vi "Metadata_Creator.vi"(7 "Frame Timestamp":u64, 8 "error in (no error)":errorcluster, 9 "Frame Index":u32, 10 "EBD Config":T2, 11 "Image Data Config":T1={"Lines of Image Data"=0, "Bytes per Even Line"=0, "Bytes per Odd Line"=0, "Image Data Type"=44, "Total Image Data Block Size"=0, "Image Data Block Offset"=0} {"Image Data Type" format="%x"}) -> (0 "error out":errorcluster, 3 "Meta Data (U8)":u8[](array[numeric]))   [LabVIEW 2020]
uses:
  ctl/Image_EBD_Config.ctl
  ctl/Image_Data_Config.ctl
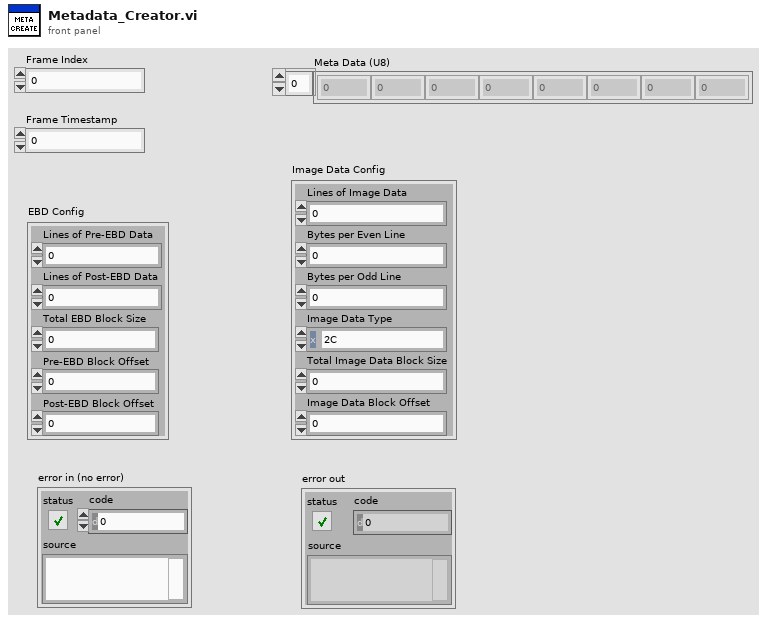
[diagram p1: front panel]
types:
  T1 = typedef "Image_Data_Config.ctl" = cluster{"Lines of Image Data":u16, "Bytes per Even Line":u16, "Bytes per Odd Line":u16, "Image Data Type":u8, "Total Image Data Block Size":u32, "Image Data Block Offset":u32}
  T2 = typedef "Image_EBD_Config.ctl" = cluster{"Lines of Pre-EBD Data":u16, "Lines of Post-EBD Data":u16, "Total EBD Block Size":u32, "Pre-EBD Block Offset ":u32, "Post-EBD Block Offset ":u32}
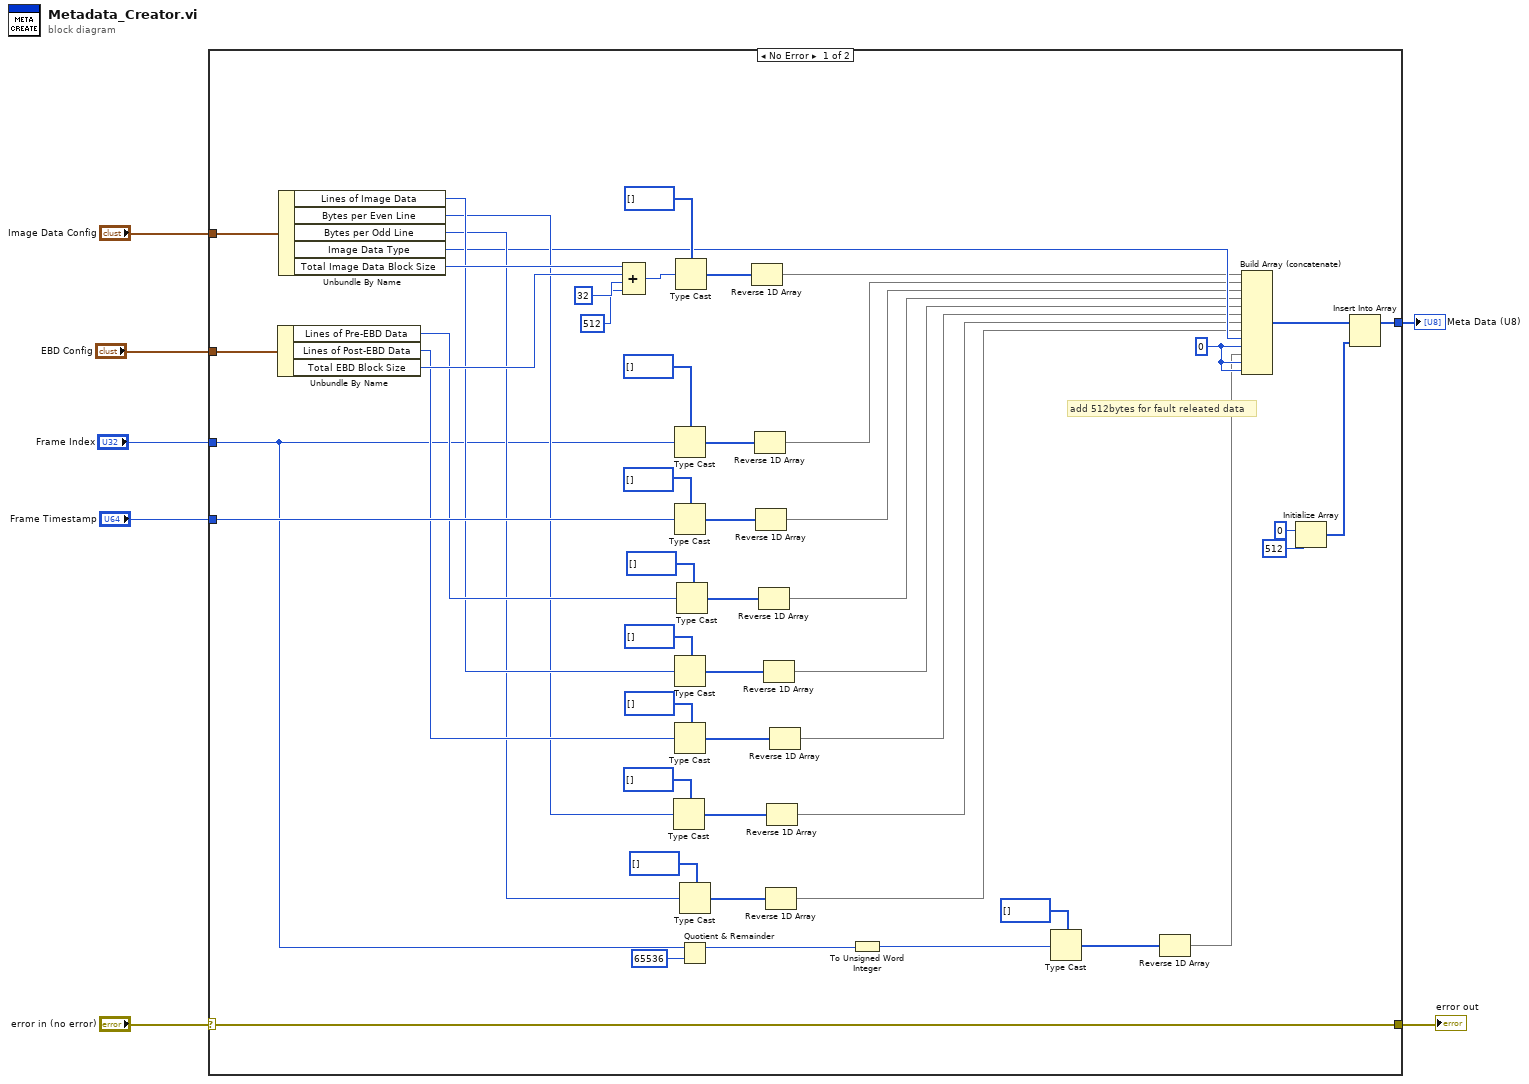
[diagram p0: block diagram]
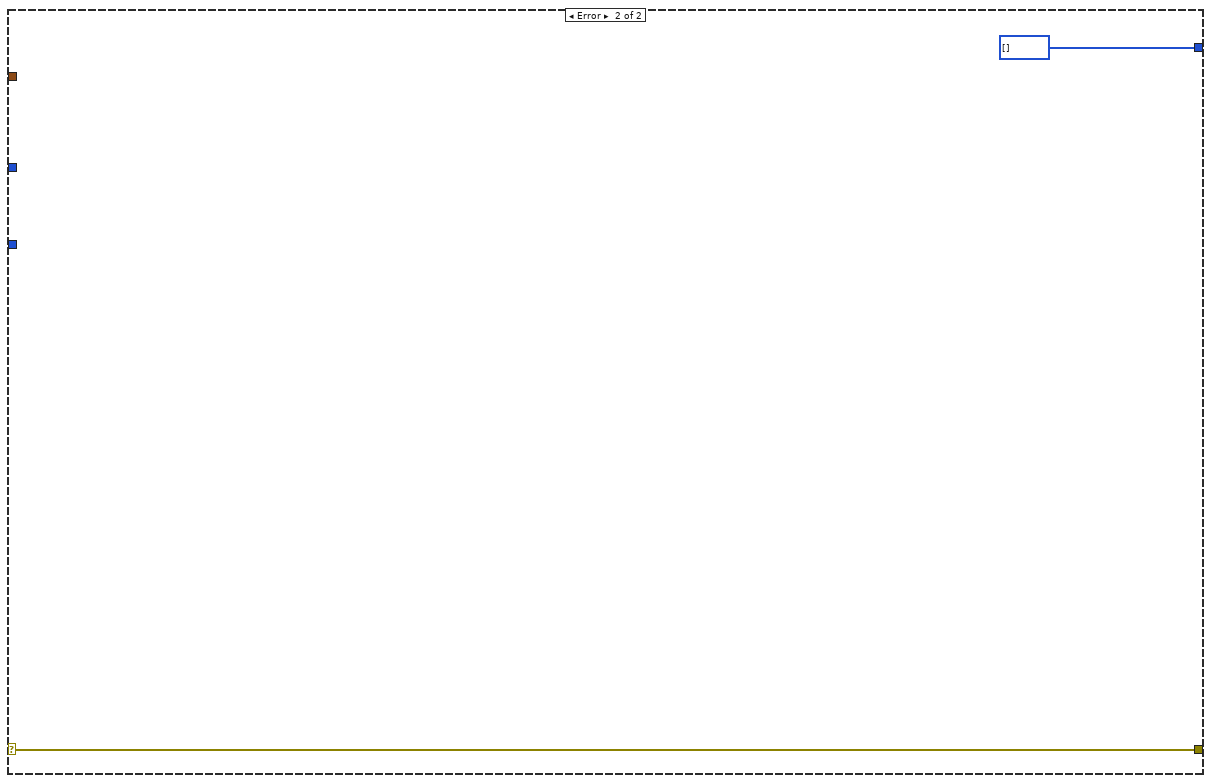
[diagram p2: hidden frame]
diagram:
  n1 = case shown="No Error" "error in (no error)" {
    selector: "error in (no error)" -> [w24 w61]
    tunnel: "Image Data Config" -> [w59 _]
    tunnel: "EBD Config" -> [w58 _]
    tunnel: "Frame Index" -> [w31 _]
    tunnel: "Frame Timestamp" -> [w50 _]
    tunnel: [w9 u8[] []] -> w2
    tunnel: [w24 w61] -> w1
    frame No Error {
      w25 = u8 0 ("element")
      # "add 512bytes for fault releated data"
      n2 = Unbundle By Name(w58) -> ("Lines of Pre-EBD Data"=w46:u16, "Lines of Post-EBD Data"=w40:u16, "Total EBD Block Size"=w56:u32)
      n3 = Unbundle By Name(w59) -> ("Lines of Image Data"=w43:u16, "Bytes per Even Line"=w37:u16, "Bytes per Odd Line"=w34:u16, "Image Data Type"=w32:u8, "Total Image Data Block Size"=w57:u32)
      n4 = Compound Arithmetic op=ADD(w57, w56, u32 32 ("value"), u32 512 ("value")) -> (w54:u32)
      n5 = Type Cast(type=u8[] [], x=w37) -> (*(type *) &x=w36:u8[])
      n6 = Type Cast(type=u8[] [], x=w31) -> (*(type *) &x=w49:u8[])
      n7 = Type Cast(type=u8[] [], x=w50) -> (*(type *) &x=w48:u8[])
      n8 = Type Cast(type=u8[] [], x=w43) -> (*(type *) &x=w42:u8[])
      n9 = Type Cast(type=u8[] [], x=w40) -> (*(type *) &x=w39:u8[])
      n10 = Type Cast(type=u8[] [], x=w54) -> (*(type *) &x=w23:u8[])
      n11 = Type Cast(type=u8[] [], x=w46) -> (*(type *) &x=w45:u8[])
      n12 = Type Cast(type=u8[] [], x=w34) -> (*(type *) &x=w33:u8[])
      n13 = Quotient & Remainder(x=w31, y=u32 65536) -> (x-y*floor(x/y)=w29:u32)  [unwired: 1 out]
      n14 = Reverse 1D Array(array=w23) -> (reversed array=w22:u8[])
      n15 = Reverse 1D Array(array=w49) -> (reversed array=w21:u8[])
      n16 = Reverse 1D Array(array=w48) -> (reversed array=w20:u8[])
      n17 = Reverse 1D Array(array=w45) -> (reversed array=w19:u8[])
      n18 = Reverse 1D Array(array=w42) -> (reversed array=w18:u8[])
      n19 = Reverse 1D Array(array=w33) -> (reversed array=w15:u8[])
      n20 = Reverse 1D Array(array=w36) -> (reversed array=w16:u8[])
      n21 = Reverse 1D Array(array=w39) -> (reversed array=w17:u8[])
      n22 = To Unsigned Word Integer(number=w29) -> (unsigned 16bit integer=w27:u16)
      n23 = Type Cast(type=u8[] [], x=w27) -> (*(type *) &x=w26:u8[])
      n24 = Reverse 1D Array(array=w26) -> (reversed array=w14:u8[])
      n25 = Build Array (concatenate)(w22, w21, w20, w19, w18, w17, w16, w15, w32, w25, w14, w25, w25) -> (w11:u8[])
      n26 = Initialize Array(u8 0 ("element"), 512 ("dimension size")) -> (w10:u8[])
      n27 = Insert Into Array(array=w11, new element=w10) -> (w9:u8[])  [unwired: 1 in]
    }
    frame Error {
    }
  }
  "error out" <- w1
  "Meta Data (U8)" <- w2
